vi "StartVITester.vi"(8 "error in (no error)":errorcluster, 11 "CommandLine":string[](array[string])) -> (0 "error out":errorcluster, 2 "test details":string)   [LabVIEW 2019]
uses:
  <vilib>/addons/_JKI Toolkits/VI Tester/VI Tester API.llb/Run Tests (Path).vi
  <vilib>/addons/_JKI Toolkits/VI Tester/VI Tester API.llb/VI Tester API.lvlib
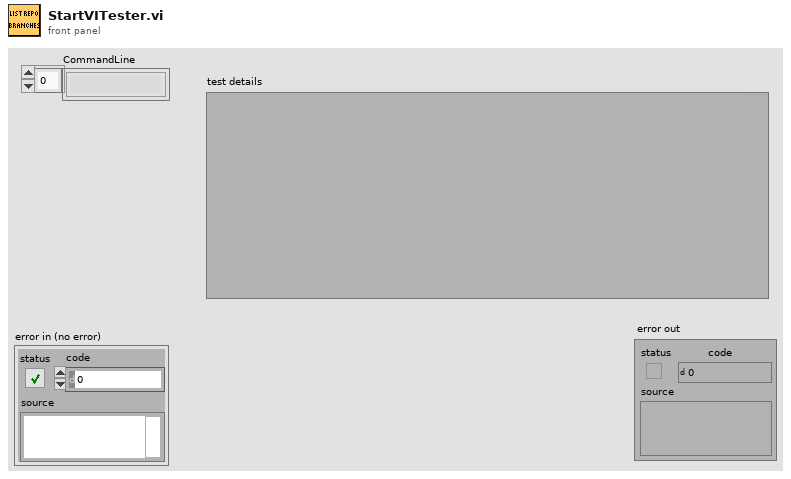
[diagram p1: front panel]
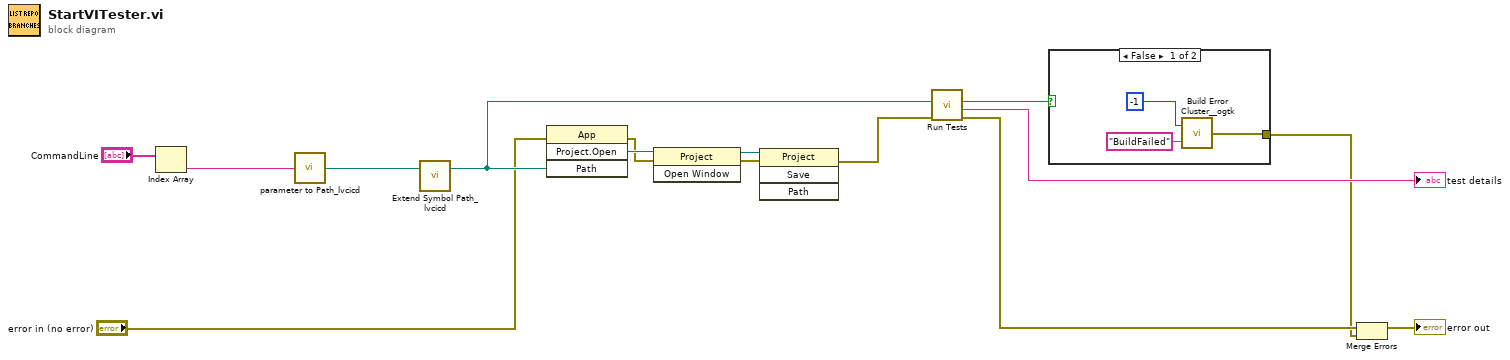
[diagram p0: block diagram]
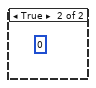
[diagram p2: hidden frame]
diagram:
  n1 = Index Array(array="CommandLine") -> (element=w13:string)  [unwired: 1 in]
  n2 = call "parameter to Path_lvcicd.vi"("String"=w13) -> ("Path"=w15:path)
  n3 = call "Extend Symbol Path_lvcicd.vi"("Symbol Path"=w15) -> ("Resolved Path"=w6:path)  [unwired: 2 in]
  n4 = invoke class="App" method="Project.Open"(error in="error in (no error)", "Path"=w6) -> (error out=w8:errorcluster, "Project:Open"=w11:refnum<vi>)  [unwired: 2 in, 2 out]
  n5 = invoke class="Project" method="Open Window"(reference=w11, error in=w8) -> (reference out=w10:refnum<vi>, error out=w9:errorcluster)  [unwired: 1 in, 1 out]
  n6 = invoke class="Project" method="Save"(reference=w10, error in=w9) -> (error out=w7:errorcluster)  [unwired: 2 in, 3 out]
  n7 = call-poly <vilib>:"Run Tests.vi"("error in (no error)"=w7, "Test Path"=w6) -> ("error out"=w3:errorcluster, "test details"=→"test details":string, "successful?"=w12:bool)  [unwired: 7 in]
  n8 = case shown="False" w12 {
    tunnel: [w16 _] -> w1
    frame False {
      n9 = call <userlib>:"Build Error Cluster__ogtk.vi"("String to Prepend to source (\"\")"="BuildFailed" ("String to Prepend to source (\"\")"), "code"=-1) -> ("error out"=w16:errorcluster)
    }
    frame True {
      (unwired) 0
    }
  }
  n10 = Merge Errors(w3, w1) -> (→"error out":errorcluster)
